vi "Power Output Version.vi"() -> ()   [LabVIEW 2011]
uses:
  SI.LIB/OGAB Version.ctl
  server/database/Fields/Field Record.ctl
  server/database/Fields/Field DataTypes.ctl
  server/database/Fields/Field NextItem.ctl
panel:
  in  "Fields":T1[](array[typedef])=[{"ixField"=0, "iSequenceOrder"=0, "sxFieldId"="C1_PIM_Power_Maximum", "sxSequenceId"="", "sDisplayName"="C1 PIM Power Maximum", "sValue"="0", "sUnits"="dBm", "nDataType"=enum."numeric", "nNextItem"=enum."Reset", "fSystem"=TRUE, "fSystemValue"=TRUE, "fRequired"=TRUE, "fSetAtTest"=TRUE, "fTestField"=TRUE, "fDeleted"=FALSE, "fIndexed"=FALSE, "fFreeList"=FALSE}, {"ixField"=0, "iSequenceOrder"=0, "sxFieldId"="C1_PIM_Power_Minimum", "sxSequenceId"="", "sDisplayName"="C1 PIM Power Minimum", "sValue"="0", "sUnits"="dBm", "nDataType"=enum."numeric", "nNextItem"=enum."Reset", "fSystem"=TRUE, "fSystemValue"=TRUE, "fRequired"=TRUE, "fSetAtTest"=TRUE, "fTestField"=TRUE, "fDeleted"=FALSE, "fIndexed"=FALSE, "fFreeList"=FALSE}, {"ixField"=0, "iSequenceOrder"=0, "sxFieldId"="C1_PWM_Power_Maximum", "sxSequenceId"="", "sDisplayName"="C1 PWM Power Maximum", "sValue"="0", "sUnits"="dBm", "nDataType"=enum."numeric", "nNextItem"=enum."Reset", "fSystem"=TRUE, "fSystemValue"=TRUE, "fRequired"=TRUE, "fSetAtTest"=TRUE, "fTestField"=TRUE, "fDeleted"=FALSE, "fIndexed"=FALSE, "fFreeList"=FALSE}, {"ixField"=0, "iSequenceOrder"=0, "sxFieldId"="C1_PWM_Power_Minimum", "sxSequenceId"="", "sDisplayName"="C1 PWM Power Minimum", "sValue"="0", "sUnits"="dBm", "nDataType"=enum."numeric", "nNextItem"=enum."Reset", "fSystem"=TRUE, "fSystemValue"=TRUE, "fRequired"=TRUE, "fSetAtTest"=TRUE, "fTestField"=TRUE, "fDeleted"=FALSE, "fIndexed"=FALSE, "fFreeList"=FALSE}, {"ixField"=0, "iSequenceOrder"=0, "sxFieldId"="C2_PIM_Power_Maximum", "sxSequenceId"="", "sDisplayName"="C2 PIM Power Maximum", "sValue"="0", "sUnits"="dBm", "nDataType"=enum."numeric", "nNextItem"=enum."Reset", "fSystem"=TRUE, "fSystemValue"=TRUE, "fRequired"=TRUE, "fSetAtTest"=TRUE, "fTestField"=TRUE, "fDeleted"=FALSE, "fIndexed"=FALSE, "fFreeList"=FALSE}, {"ixField"=0, "iSequenceOrder"=0, "sxFieldId"="C2_PIM_Power_Minimum", "sxSequenceId"="", "sDisplayName"="C2 PIM Power Minimum", "sValue"="0", "sUnits"="dBm", "nDataType"=enum."numeric", "nNextItem"=enum."Reset", "fSystem"=TRUE, "fSystemValue"=TRUE, "fRequired"=TRUE, "fSetAtTest"=TRUE, "fTestField"=TRUE, "fDeleted"=FALSE, "fIndexed"=FALSE, "fFreeList"=FALSE}, {"ixField"=0, "iSequenceOrder"=0, "sxFieldId"="C2_PWM_Power_Maximum", "sxSequenceId"="", "sDisplayName"="C2 PWM Power Maximum", "sValue"="0", "sUnits"="dBm", "nDataType"=enum."numeric", "nNextItem"=enum."Reset", "fSystem"=TRUE, "fSystemValue"=TRUE, "fRequired"=TRUE, "fSetAtTest"=TRUE, "fTestField"=TRUE, "fDeleted"=FALSE, "fIndexed"=FALSE, "fFreeList"=FALSE}, {"ixField"=0, "iSequenceOrder"=0, "sxFieldId"="C2_PWM_Power_Minimum", "sxSequenceId"="", "sDisplayName"="C2 PWM Power Minimum", "sValue"="0", "sUnits"="dBm", "nDataType"=enum."numeric", "nNextItem"=enum."Reset", "fSystem"=TRUE, "fSystemValue"=TRUE, "fRequired"=TRUE, "fSetAtTest"=TRUE, "fTestField"=TRUE, "fDeleted"=FALSE, "fIndexed"=FALSE, "fFreeList"=FALSE}, {"ixField"=0, "iSequenceOrder"=0, "sxFieldId"="Calibration_Status", "sxSequenceId"="", "sDisplayName"="Calibration Status", "sValue"="0", "sUnits"="", "nDataType"=enum."numeric", "nNextItem"=enum."Reset", "fSystem"=TRUE, "fSystemValue"=TRUE, "fRequired"=TRUE, "fSetAtTest"=TRUE, "fTestField"=TRUE, "fDeleted"=FALSE, "fIndexed"=FALSE, "fFreeList"=FALSE}, {"ixField"=0, "iSequenceOrder"=0, "sxFieldId"="Cycles", "sxSequenceId"="", "sDisplayName"="Cycles", "sValue"="0", "sUnits"="", "nDataType"=enum."numeric", "nNextItem"=enum."Reset", "fSystem"=TRUE, "fSystemValue"=TRUE, "fRequired"=TRUE, "fSetAtTest"=TRUE, "fTestField"=TRUE, "fDeleted"=FALSE, "fIndexed"=FALSE, "fFreeList"=FALSE}, {"ixField"=0, "iSequenceOrder"=0, "sxFieldId"="DUT_Port", "sxSequenceId"="", "sDisplayName"="DUT Port", "sValue"="Port 1\tPort 1\tPort 2", "sUnits"="", "nDataType"=enum."list", "nNextItem"=enum."Reset", "fSystem"=TRUE, "fSystemValue"=TRUE, "fRequired"=TRUE, "fSetAtTest"=TRUE, "fTestField"=TRUE, "fDeleted"=FALSE, "fIndexed"=FALSE, "fFreeList"=FALSE}, {"ixField"=0, "iSequenceOrder"=0, "sxFieldId"="Frequency_Type", "sxSequenceId"="", "sDisplayName"="Frequency Type", "sValue"="Band Edges\tBand Edges\tCustom", "sUnits"="", "nDataType"=enum."list", "nNextItem"=enum."Reset", "fSystem"=TRUE, "fSystemValue"=TRUE, "fRequired"=TRUE, "fSetAtTest"=TRUE, "fTestField"=TRUE, "fDeleted"=FALSE, "fIndexed"=FALSE, "fFreeList"=FALSE}, {"ixField"=0, "iSequenceOrder"=0, "sxFieldId"="IM_Mode", "sxSequenceId"="", "sDisplayName"="IM Mode", "sValue"="Reverse\tReverse\tForward\tAuxilary", "sUnits"="", "nDataType"=enum."list", "nNextItem"=enum."Reset", "fSystem"=TRUE, "fSystemValue"=TRUE, "fRequired"=TRUE, "fSetAtTest"=TRUE, "fTestField"=TRUE, "fDeleted"=FALSE, "fIndexed"=FALSE, "fFreeList"=FALSE}, {"ixField"=0, "iSequenceOrder"=0, "sxFieldId"="Instrument_Calibration_Date", "sxSequenceId"="", "sDisplayName"="Instrument Calibration Date", "sValue"="0", "sUnits"="", "nDataType"=enum."timestamp", "nNextItem"=enum."Reset", "fSystem"=TRUE, "fSystemValue"=TRUE, "fRequired"=TRUE, "fSetAtTest"=TRUE, "fTestField"=TRUE, "fDeleted"=FALSE, "fIndexed"=FALSE, "fFreeList"=FALSE}, {"ixField"=0, "iSequenceOrder"=0, "sxFieldId"="Instrument_Calibration_Due_Date", "sxSequenceId"="", "sDisplayName"="Instrument Calibration Due Date", "sValue"="0", "sUnits"="", "nDataType"=enum."timestamp", "nNextItem"=enum."Reset", "fSystem"=TRUE, "fSystemValue"=TRUE, "fRequired"=TRUE, "fSetAtTest"=TRUE, "fTestField"=TRUE, "fDeleted"=FALSE, "fIndexed"=FALSE, "fFreeList"=FALSE}, {"ixField"=0, "iSequenceOrder"=0, "sxFieldId"="Instrument_Driver", "sxSequenceId"="", "sDisplayName"="Instrument Driver", "sValue"="", "sUnits"="", "nDataType"=enum."text", "nNextItem"=enum."Reset", "fSystem"=TRUE, "fSystemValue"=TRUE, "fRequired"=TRUE, "fSetAtTest"=TRUE, "fTestField"=TRUE, "fDeleted"=FALSE, "fIndexed"=FALSE, "fFreeList"=FALSE}, {"ixField"=0, "iSequenceOrder"=0, "sxFieldId"="Instrument_Name", "sxSequenceId"="", "sDisplayName"="Instrument Name", "sValue"="", "sUnits"="", "nDataType"=enum."text", "nNextItem"=enum."Reset", "fSystem"=TRUE, "fSystemValue"=TRUE, "fRequired"=TRUE, "fSetAtTest"=TRUE, "fTestField"=TRUE, "fDeleted"=FALSE, "fIndexed"=FALSE, "fFreeList"=FALSE}, {"ixField"=0, "iSequenceOrder"=0, "sxFieldId"="Instrument_Serial_Number", "sxSequenceId"="", "sDisplayName"="Instrument Serial Number", "sValue"="", "sUnits"="", "nDataType"=enum."text", "nNextItem"=enum."Reset", "fSystem"=TRUE, "fSystemValue"=TRUE, "fRequired"=TRUE, "fSetAtTest"=TRUE, "fTestField"=TRUE, "fDeleted"=FALSE, "fIndexed"=FALSE, "fFreeList"=FALSE}, {"ixField"=0, "iSequenceOrder"=0, "sxFieldId"="Instrument_Type", "sxSequenceId"="", "sDisplayName"="Instrument Type", "sValue"="", "sUnits"="", "nDataType"=enum."text", "nNextItem"=enum."Reset", "fSystem"=TRUE, "fSystemValue"=TRUE, "fRequired"=TRUE, "fSetAtTest"=TRUE, "fTestField"=TRUE, "fDeleted"=FALSE, "fIndexed"=FALSE, "fFreeList"=FALSE}, {"ixField"=0, "iSequenceOrder"=0, "sxFieldId"="Minimum_Power", "sxSequenceId"="", "sDisplayName"="Minimum Power", "sValue"="44", "sUnits"="dBm", "nDataType"=enum."numeric", "nNextItem"=enum."Reset", "fSystem"=TRUE, "fSystemValue"=TRUE, "fRequired"=TRUE, "fSetAtTest"=TRUE, "fTestField"=TRUE, "fDeleted"=FALSE, "fIndexed"=FALSE, "fFreeList"=FALSE}, {"ixField"=0, "iSequenceOrder"=0, "sxFieldId"="Pad_Model_Number", "sxSequenceId"="", "sDisplayName"="Pad Model Number", "sValue"="", "sUnits"="", "nDataType"=enum."text", "nNextItem"=enum."Reset", "fSystem"=TRUE, "fSystemValue"=TRUE, "fRequired"=TRUE, "fSetAtTest"=TRUE, "fTestField"=TRUE, "fDeleted"=FALSE, "fIndexed"=FALSE, "fFreeList"=FALSE}, {"ixField"=0, "iSequenceOrder"=0, "sxFieldId"="Pad_Serial_Number", "sxSequenceId"="", "sDisplayName"="Pad Serial Number", "sValue"="", "sUnits"="", "nDataType"=enum."text", "nNextItem"=enum."Reset", "fSystem"=TRUE, "fSystemValue"=TRUE, "fRequired"=TRUE, "fSetAtTest"=TRUE, "fTestField"=TRUE, "fDeleted"=FALSE, "fIndexed"=FALSE, "fFreeList"=FALSE}]
  in  "QuickMode":i32
  in  "DriverTypes":string[](array[string])=["PIM", "PWM"]
  in  "Description":string="This test will perform Passive Intermodulation Power Output testing using a Passive Intermodulation (PIM) analyzer and a Power Meter (PWM)."
  in  "Version":T4={"Version"="6.3", "Build Number"=12, "Build Date/Time"=3440694548.419435} {"Build Date/Time" format="%<%X\n%x>T"}
  # "Note: The version\nglobal is set during\nbuild.  Don't change\nor rename this variable"
  # "This is an array of fields\nto be added to the DB if\nthis test is placed into a\ntest sequence."
  # "Add a description for this\ntest before building"
  # "Add a list of driver types\n(e.g., PIM,...) required\nby the test (can be empty)"
  # "QuickMode:\n0 = Supported (OFF By Default)\n1 = Supported (ON By Default)\n2 = Not Supported"
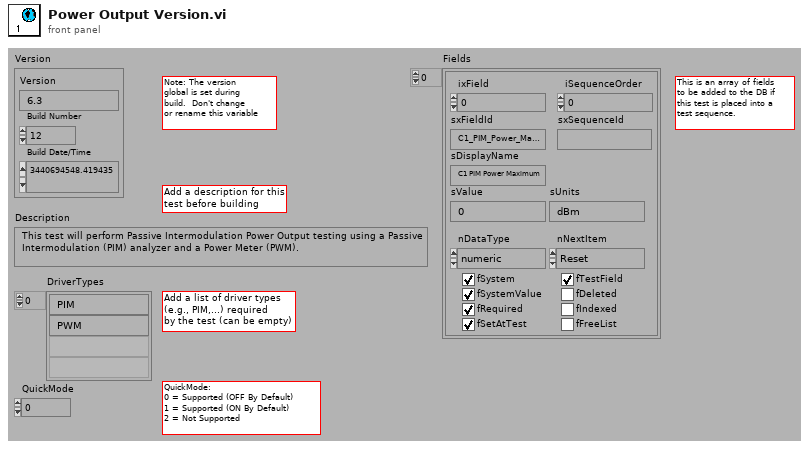
[diagram p1: front panel]
types:
  T1 = typedef "Field Record.ctl" = cluster{"ixField":i32, "iSequenceOrder":i32, "sxFieldId":string, "sxSequenceId":string, "sDisplayName":string, "sValue":string, "sUnits":string, "nDataType":T2, "nNextItem":T3, "fSystem":bool, "fSystemValue":bool, "fRequired":bool, "fSetAtTest":bool, "fTestField":bool, "fDeleted":bool, "fIndexed":bool, "fFreeList":bool}
  T2 = typedef "Field DataTypes.ctl" = enum32{"text", "numeric", "list", "timestamp", "boolean"}
  T3 = typedef "Field NextItem.ctl" = enum32{"Reset", "Retain", "Auto-Increment"}
  T4 = typedef "OGAB Version.ctl" = cluster{"Version":string, "Build Number":u32, "Build Date/Time":dbl}
diagram:
